vi "get_lights.vi"(10 "Selector":enum16{"Handle lights", "Tip lights"}(ring), 11 "ASAP data":sgl[][](array[numeric])) -> (3 "Light positions":T1 format="%#.1f")   [LabVIEW 2013]
uses:
  probe_calibration.ctl
panel:
  # "0 Is handle lights, 1 is tip"
  # "Select tip or handle lights from 6x3 array of ASAP data."
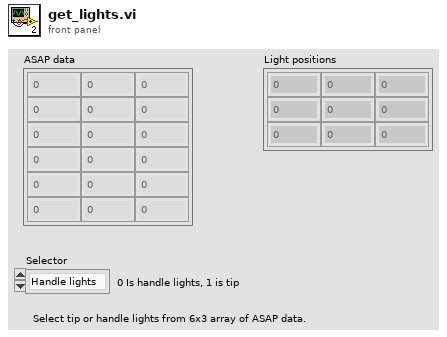
[diagram p1: front panel]
types:
  T1 = typedef "probe_calibration.ctl" = sgl[][]
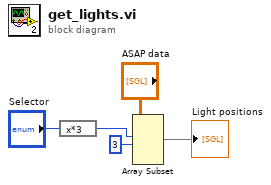
[diagram p0: block diagram]
diagram:
  n1 = expression code="x*3"("Selector") -> (w4:enum16{"Handle lights", "Tip lights"})
  n2 = Array Subset(array="ASAP data", index (row)=w4, length (row)=3 ("length")) -> (→"Light positions":sgl[][])  [unwired: 2 in]
